vi "Problem2.2.vi"() -> ()   [LabVIEW 2019]
panel:
  out "Timer Done":bool
  in  "Wait Time (Seconds)":dbl=4.0
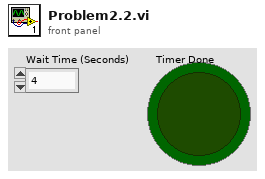
[diagram p1: front panel]
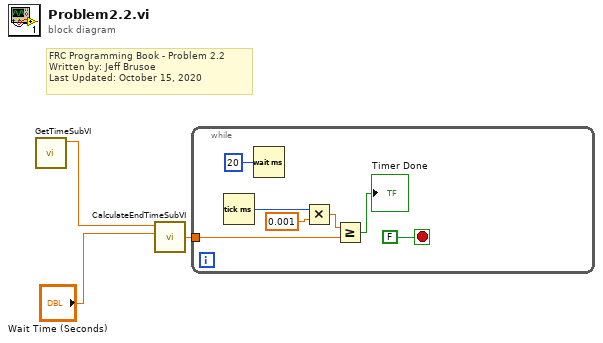
[diagram p0: block diagram]
diagram:
  # "FRC Programming Book - Problem 2.2\nWritten by: Jeff Brusoe\nLast Updated: October 15, 2020"
  n1 = call "GetTimeSubVI.vi"() -> ("Seconds"=w1:dbl)  [unwired: 11 in]
  n2 = call "CalculateEndTimeSubVI.vi"("Wait Time (Seconds)"="Wait Time (Seconds)", "Current Time (Seconds)"=w1) -> ("End Time (Seconds)"=w2:dbl)  [unwired: 9 in]
  n3 = while {
    tunnel: w2 -> [w10]
    stop <- FALSE stop-if-true
    n4 = Tick Count (ms)() -> (millisecond timer value=w7:u32)
    n5 = Wait (ms)(milliseconds to wait=u32 20) -> ()  [unwired: 1 out]
    n6 = Multiply(x=w7, y=0.001) -> (x*y=w6:dbl)
    n7 = Greater Or Equal?(x=w6, y=w10) -> (x >= y?=→"Timer Done":bool)
  }
